vi "Setup MQTT Channel.vi"(4 "Excluded (None)":refnum<class "Message.lvclass">[](array[class]), 5 "MQTT Setup":T3, 6 "Included (All)":refnum<class "Message.lvclass">[](array[class]), 7 "Emit Status Messages (F)":bool, 8 "error in (no error)":errorcluster, 9 "Topic Prefix":string, 10 "Connection Configuration":refnum<class "Connection.lvclass">, 11 "AF MQTT Message Channel in":refnum<class "AF MQTT Message Channel.lvclass">) -> (0 "error out":errorcluster, 3 "AF MQTT Message Channel out":refnum<class "AF MQTT Message Channel.lvclass">)   [LabVIEW 2020, in "AF MQTT Channel.lvlib" / "AF MQTT Message Channel.lvclass"]
uses:
  AF MQTT Message Channel.lvclass
  <vilib>/LabVIEW Open Source Project/MQTT Connection/MQTT_Connection/Connection/Connection.lvclass
  <vilib>/LabVIEW Open Source Project/MQTT Control Packets/Control Packets/ControlPacket/QualityOfService -- enum.ctl
  <vilib>/LabVIEW Open Source Project/MQTT Control Packets/Control Packets/CONNECT/ConnectFlags -- cluster.ctl
  AF MQTT Message Channel.lvclass/AF MQTT Message Channel.ctl
  Actor Pub Sub Channels/Pub Sub Message Channel/Pub Sub Message Channel.lvclass
  C:/Users/Simon/Documents/GitHub/LV-Actor-Pub-Sub/Source/Actor Pub Sub Channels/Pub Sub Message Channel/Pub Sub Message Channel.lvclass
  C:/Users/Simon/Documents/GitHub/LV-Actor-Pub-Sub/Source/AF MQTT Channel/AF MQTT Message Channel/AF MQTT Message Channel.lvclass
  <vilib>/LabVIEW Open Source Project/MQTT Control Packets/Control Packets/ControlPacket/ControlPacket.lvclass
  <vilib>/LabVIEW Open Source Project/MQTT Control Packets/Control Packets/CONNECT/CONNECT.lvclass
  <vilib>/ActorFramework/Message/Message.lvclass
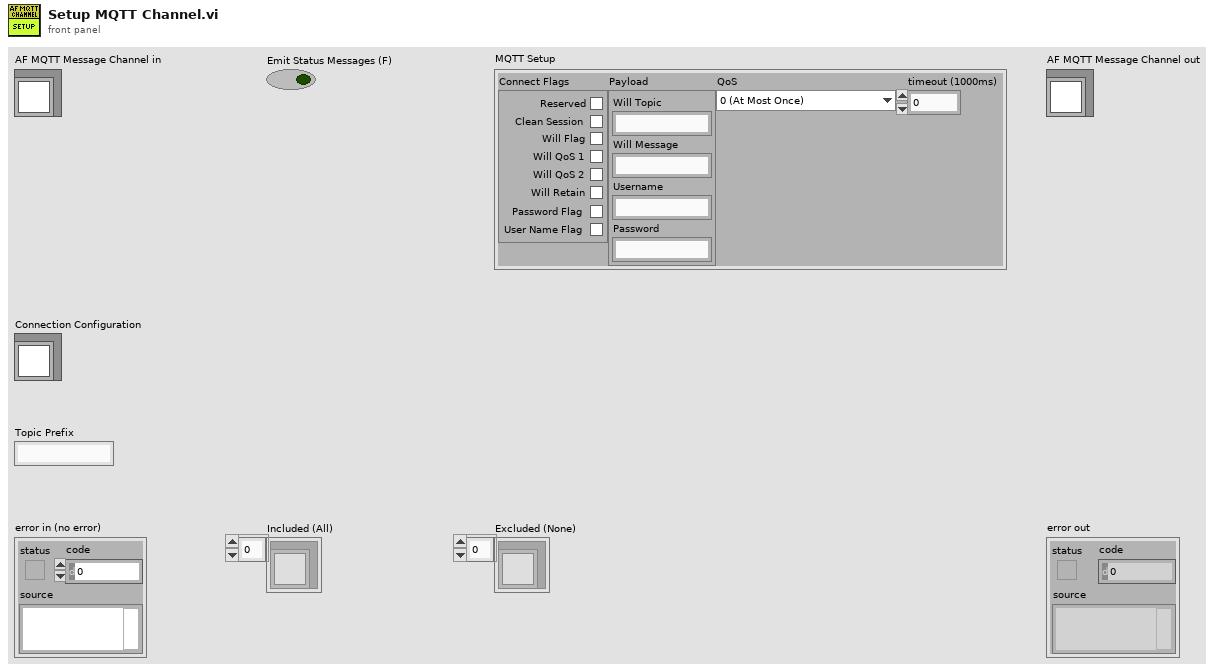
[diagram p1: front panel]
types:
  T1 = typedef "MQTT_Control_Packets.lvlib/CONNECT.lvclass/ConnectFlags -- cluster.ctl" = cluster{"Reserved":bool, "Clean Session":bool, "Will Flag":bool, "Will QoS 1":bool, "Will QoS 2":bool, "Will Retain":bool, "Password Flag":bool, "User Name Flag":bool}
  T2 = typedef "MQTT_Control_Packets.lvlib/ControlPacket.lvclass/QualityOfService -- enum.ctl" = enum16{"0 (At Most Once)", "1 (At Least Once)", "2 (Exactly Once)"}
  T3 = cluster{"Connect Flags":T1, "Payload":cluster{"Will Topic":string, "Will Message":string, "Username":string, "Password":string}, "QoS":T2, "timeout (1000ms)":i32}
  T4 = cluster{"Will Topic":string, "Will Message":string, "Username":string, "Password":string}
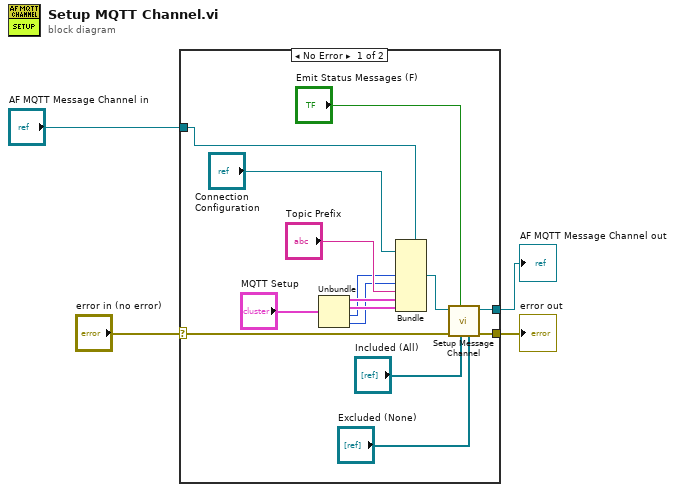
[diagram p0: block diagram]
diagram:
  n1 = case shown="No Error" "error in (no error)" {
    selector: "error in (no error)" -> [w18 w21]
    tunnel: [w13 w21] -> w3
    tunnel: [w11 w20] -> w1
    tunnel: "AF MQTT Message Channel in" -> [w19 w20]
    frame No Error {
      n2 = Unbundle("MQTT Setup") -> ("Connect Flags"=w15:T1, "Payload"=w14:T4, "QoS"=w10:T2, "timeout (1000ms)"=w9:i32)
      n3 = Bundle(cluster=w19, "Connection Configuration", w10, w9, "Topic Prefix", w15, w14) -> (w12:refnum<class "AF MQTT Message Channel.lvclass">)  [unwired: 3 in]
      n4 = call "Setup Message Channel.vi"("Excluded (None)"="Excluded (None)", "Included (All)"="Included (All)", "Emit Status Messages (F)"="Emit Status Messages (F)", "error in (no error)"=w18, "Pub Sub Message Channel in"=w12) -> ("error out"=w13:errorcluster, "Pub Sub Message Channel out"=w11:refnum<class "AF MQTT Message Channel.lvclass">)  [unwired: 5 in]
    }
    frame Error {
    }
  }
  "error out" <- w3
  "AF MQTT Message Channel out" <- w1
